vi "MethodSignatureDialogvi.vi"() -> (2 "Cancelled":bool)   [LabVIEW 2014, in "ClassWriterNative.lvclass"]
uses:
  <resource>/Framework/Providers/Open_GDS/ClassProviders/Provider_LvNativeClass/ClassWriterNative_class/ClassWriterNative.lvclass
  <resource>/Framework/Providers/Open_GDS/SubVIs/GOOP_HelpButton.ctl
panel:
  in  "_HelpCreateSignature":T1
  in  "_UpdateSignature":bool caption="Update this signature"
  in  "_InsertTag":bool caption="Insert tag"
  out "_TagPreview":string caption="Tag preview"
  in  "_SelectTagToAdd":T2(ring) caption="Select a tag to a cursor"
  in  "_SignatureName":string caption="Signature name"
  in  "_ModifySignature":bool caption="Modify signature"
  in  "_RemoveSignature":bool caption="Remove signature"
  in  "_Cancel":bool caption="Cancel"
  in  "_Done":bool caption="Done"
  in  "_AddSignature":bool caption="Add this signature"
  in  "_Signatures":i32[](listbox) caption="Signatures"
  in  "_SignatureText":string caption="Signature text"
  out "error out":errorcluster
  in  "error in":errorcluster
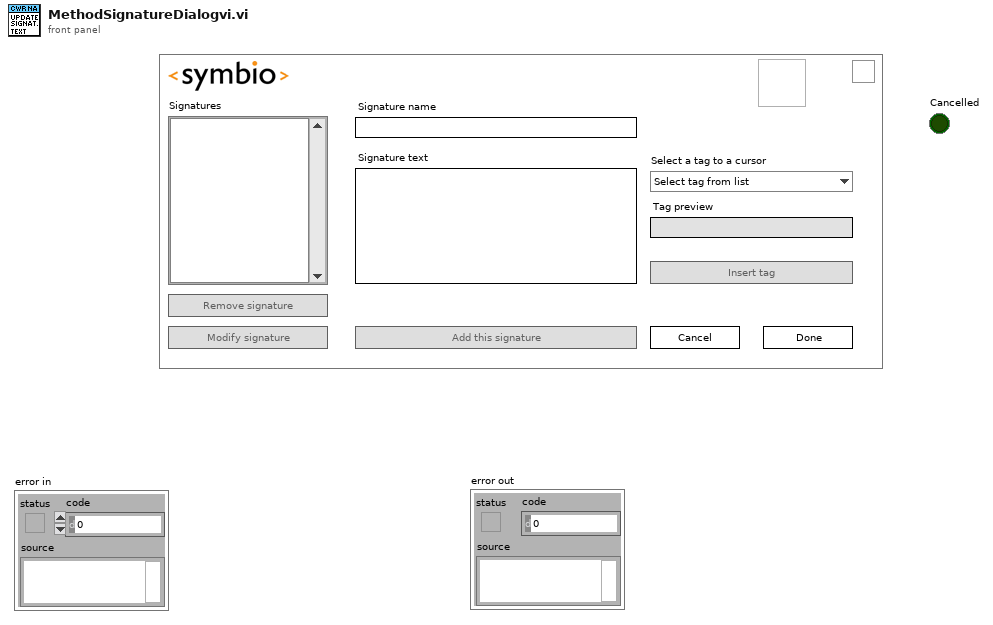
[diagram p1: front panel]
types:
  T1 = typedef "GOOP_HelpButton.ctl" = bool
  T2 = enum16{"Select tag from list", "<Date>", "<DateTime>", "<User>", "<LvVersion>"}
  T3 = cluster{"Cancelled":bool, "SignatureName":string[], "SignatureText":string[], "Current":i32}
  T4 = cluster{"SignatureName":string[], "SignatureText":string[], "Current":i32}
  T5 = cluster{"SignatureName":string[], "SignatureText":string[], i32}
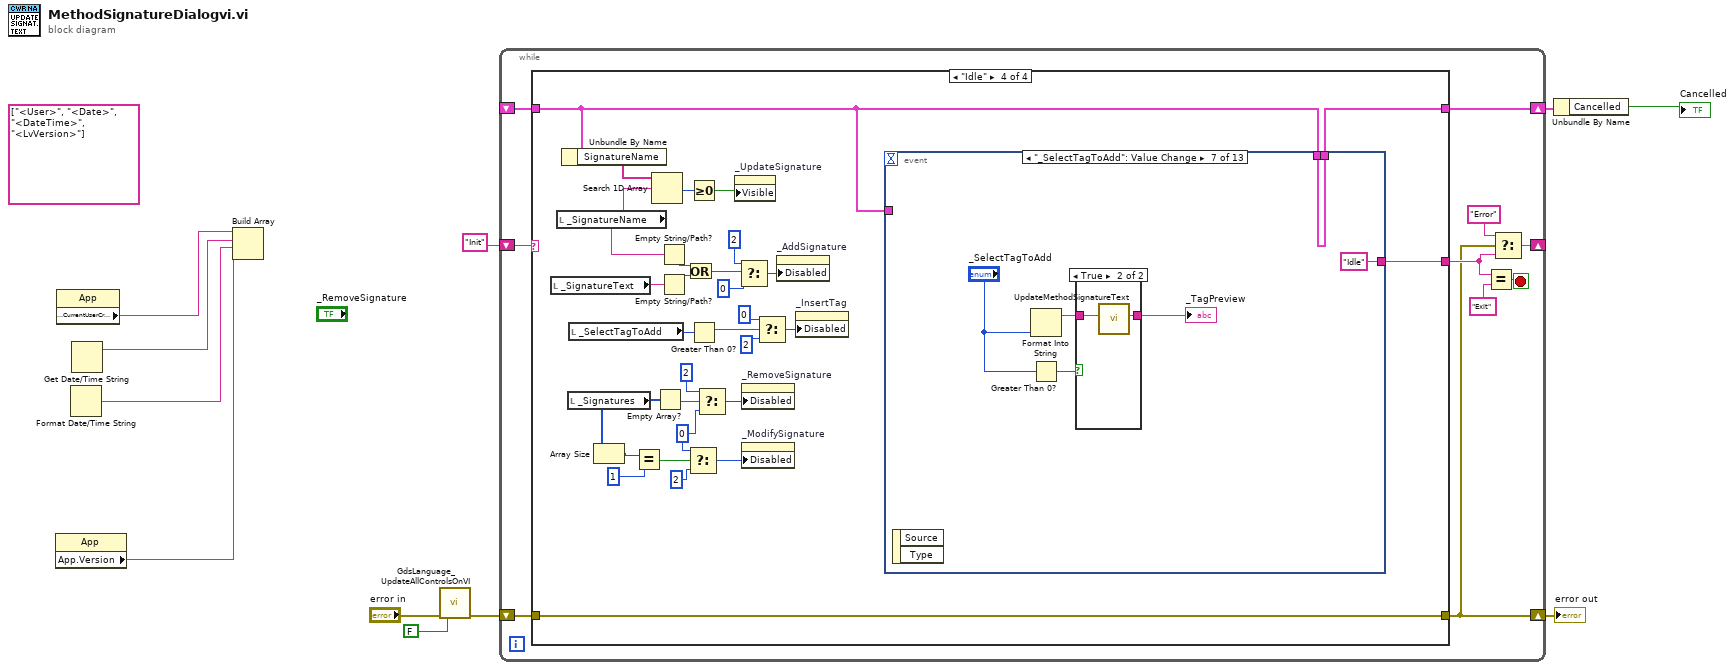
[diagram p0: block diagram]
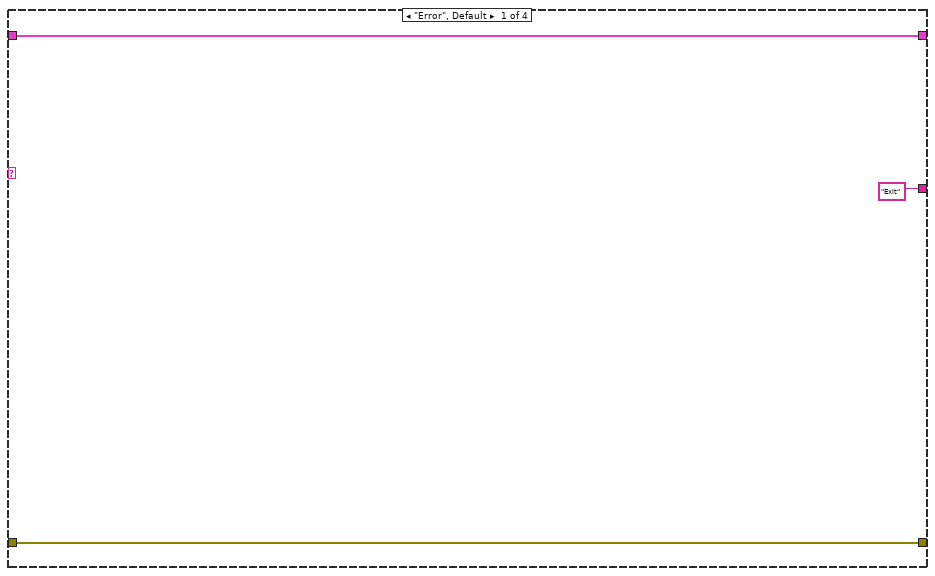
[diagram p2: hidden frame]
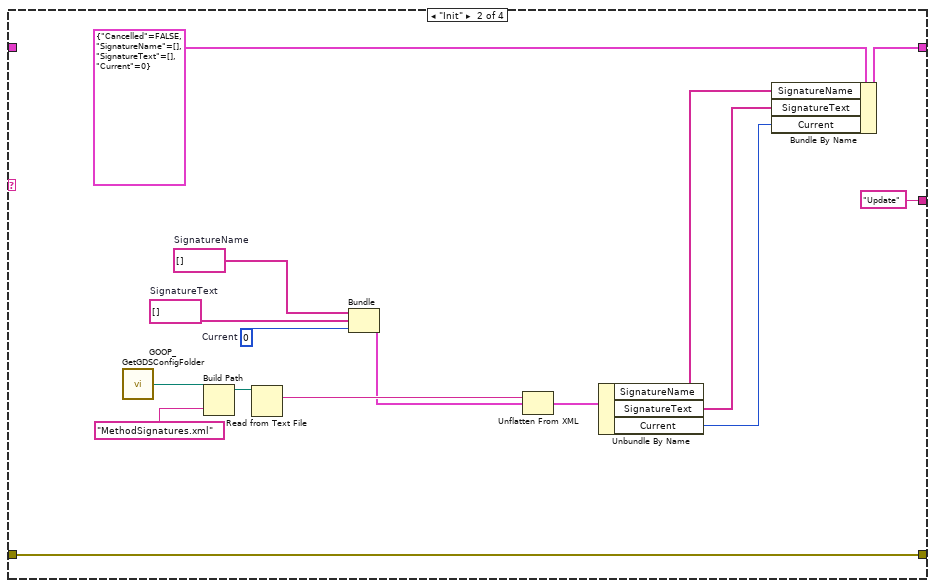
[diagram p3: hidden frame]
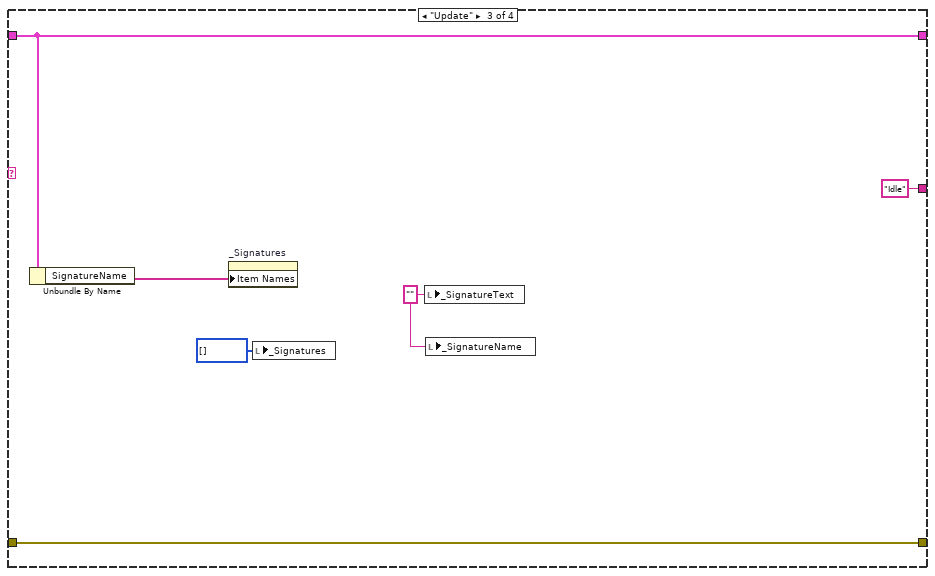
[diagram p4: hidden frame]
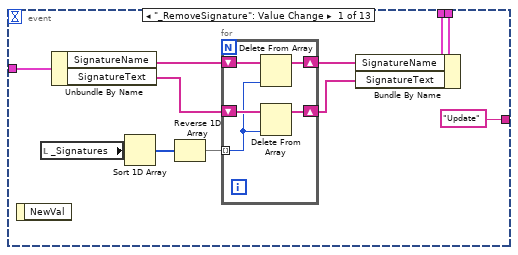
[diagram p5: hidden frame]
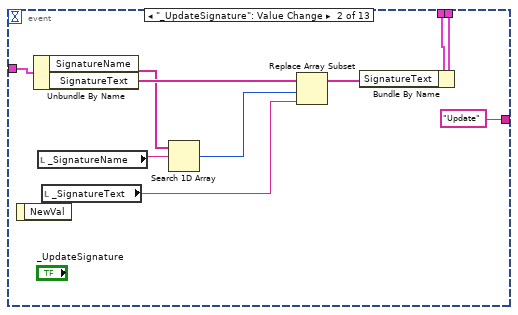
[diagram p6: hidden frame]
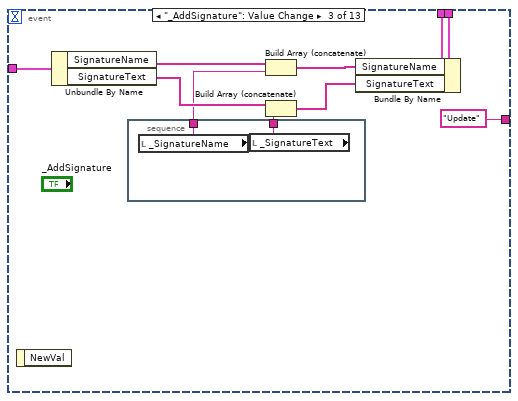
[diagram p7: hidden frame]
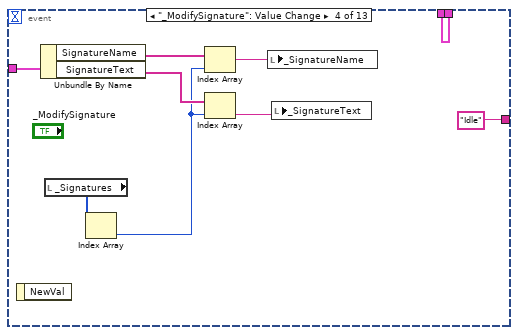
[diagram p8: hidden frame]
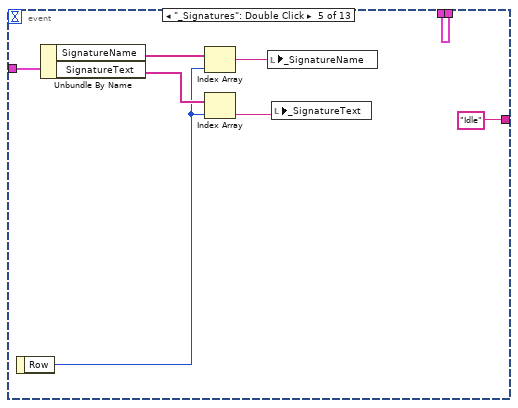
[diagram p9: hidden frame]
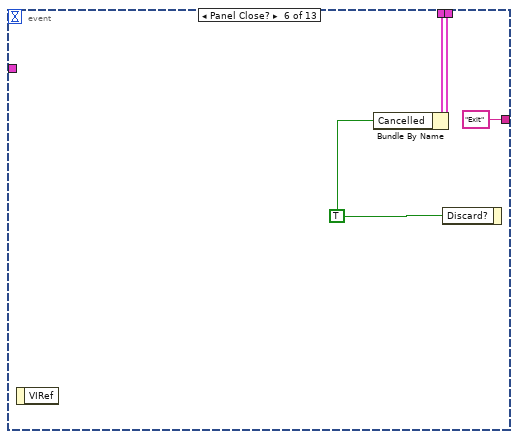
[diagram p10: hidden frame]
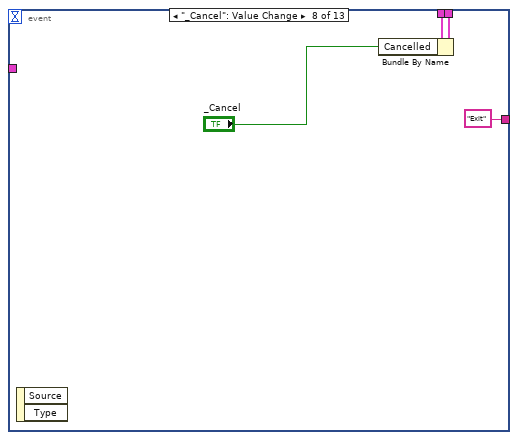
[diagram p12: hidden frame]
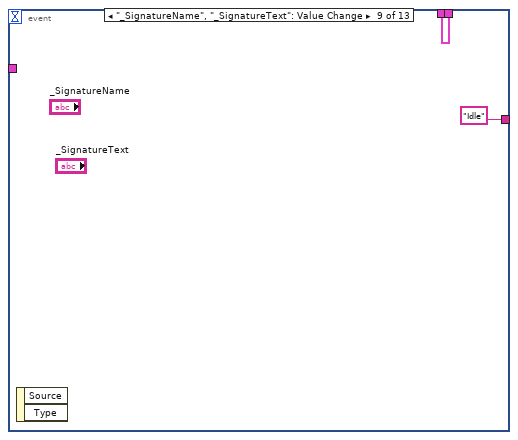
[diagram p13: hidden frame]
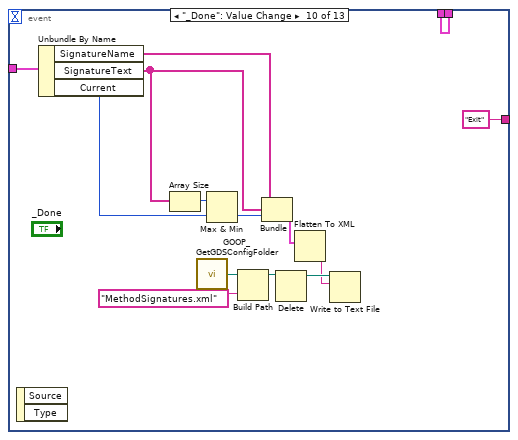
[diagram p14: hidden frame]
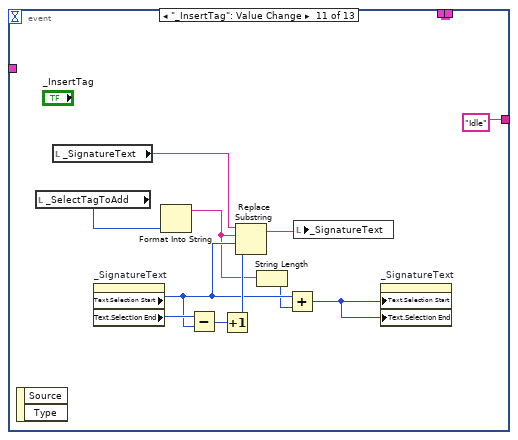
[diagram p15: hidden frame]
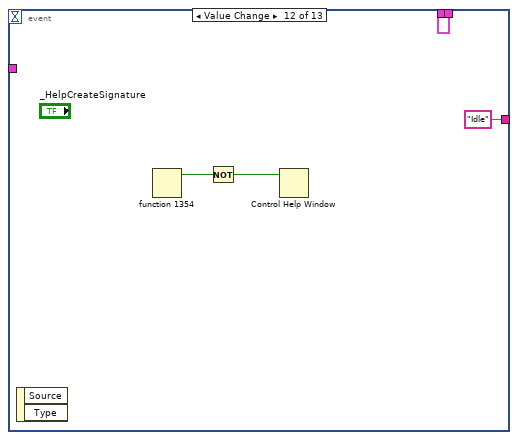
[diagram p16: hidden frame]
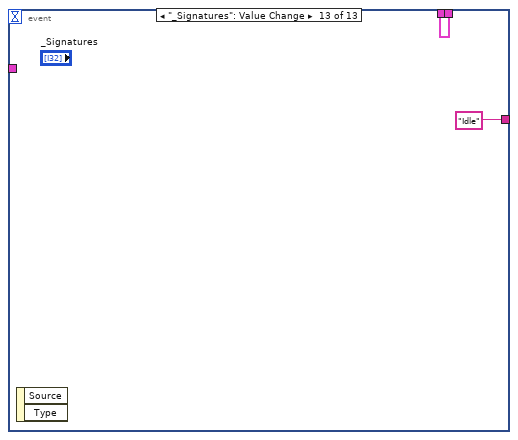
[diagram p17: hidden frame]
diagram:
  (unwired) string[] ["<User>", "<Date>", "<DateTime>", "<LvVersion>"]
  n1 = property class="App"() -> ("App.Version"=w8:string)  [unwired: 2 in, 2 out]
  n2 = property class="App"() -> ("App.CurrentUserCredential"=w11:string)  [unwired: 2 in, 2 out]
  n3 = Format Date/Time String() -> (date/time string=w9:string)  [unwired: 3 in]
  n4 = Get Date/Time String() -> (date string=w10:string)  [unwired: 3 in, 1 out]
  n5 = Build Array(w11, w10, w9, w8) -> ()  [unwired: 1 out]
  n6 = call <resource>:"GdsLanguage_UpdateAllControlsOnVI.vi"("error in (no error)"="error in", "CreateLanguageFile(Use this to create a languageFile)"=FALSE) -> ("error out"=w2:errorcluster)  [unwired: 16 in, 1 out]
  n7 = while {
    shift-right: [w14] -> w4
    shift-left: w2 -> [w21]
    shift-right: [w19] -> _
    shift-left: "Init" -> [w20]
    shift-right: [w13] -> w6
    shift-left: _ -> [w12]
    stop <- w18 stop-if-true
    n8 = case shown="\"Idle\"" w20 {
      tunnel: w21 -> [w24 w39 w44 w74]
      tunnel: [w24 w39 w44 w74] -> w14
      tunnel: ["Exit" "Update" "Idle" w75] -> w15
      tunnel: [w22 w37 w45 w76] -> w13
      tunnel: w12 -> [w22 _ w45 w63]
      frame "Error", Default {
      }
      frame "Init" {
        w32 = string[] []  # SignatureText
        w33 = string[] []  # SignatureName
        w30 = 0  # Current
        n9 = call <resource>:"GOOP_GetGDSConfigFolder.vi"() -> ("GDSFolderPath"=w36:path)
        n10 = Build Path(base path=w36, name or relative path="MethodSignatures.xml") -> (appended path=w35:path)
        n11 = Read from Text File(file (use dialog)=w35) -> (text=w34:string)  [unwired: 3 in, 3 out]
        n12 = Bundle("SignatureName"=w33, "SignatureText"=w32, "Current"=w30) -> (w31:T4)  [unwired: 1 in]
        n13 = Unflatten From XML(xml string=w34, type=w31) -> (value=w29:T4)  [unwired: 1 in, 1 out]
        n14 = Unbundle By Name(w29) -> ("SignatureName"=w28:string[], "SignatureText"=w27:string[], "Current"=w26:i32)
        n15 = Bundle By Name(cluster=T3 {"Cancelled"=FALSE, "SignatureName"=[], "SignatureText"=[], "Current"=0}, "SignatureName"=w28, "SignatureText"=w27, "Current"=w26) -> (w37:T3)
      }
      frame "Update" {
        w41 = "" ("_SignatureText")
        n16 = Unbundle By Name(w45) -> ("SignatureName"=w43:string[])
        n17 = property on="_Signatures" class="LstBox (strict)"("Item Names"=w43) -> ()  [unwired: 2 in, 2 out]
        n18 = local write "_Signatures"(i32[] [] ("_Signatures")) -> ()
        n19 = local write "_SignatureText"(w41) -> ()
        n20 = local write "_SignatureName"(w41) -> ()
      }
      frame "Idle" {
        w66 = u8 0 ("f")
        n21 = local read "_SignatureText"() -> (w58:string)
        n22 = local read "_SignatureName"() -> (w59:string)
        n23 = Unbundle By Name(w63) -> ("SignatureName"=w62:string[])
        n24 = local read "_Signatures"() -> (w70:i32[])
        n25 = local read "_SelectTagToAdd"() -> (w51:T2)
        n26 = Array Size(array=w70) -> (size(s)=w69:i32)
        n27 = Equal?(x=w69, y=1) -> (x = y?=w65:bool)
        n28 = Search 1D Array(1D array=w62, element=w59) -> (index of element=w61:i32)  [unwired: 1 in]
        n29 = Empty Array?(array=w70) -> (empty?=w73:bool)
        n30 = Empty String/Path?(string/path=w59) -> (empty?=w57:bool)
        n31 = Empty String/Path?(string/path=w58) -> (empty?=w56:bool)
        n32 = Or(x=w57, y=w56) -> (x .or. y?=w53:bool)
        n33 = Select(t=w66, s=w65, f=u8 2) -> (s? t:f=w64:u8)
        n34 = Greater Or Equal To 0?(x=w61) -> (x >= 0?=w60:bool)
        n35 = Greater Than 0?(x=w51) -> (x > 0?=w49:bool)
        n36 = Select(t=u8 2 ("Disabled"), s=w73, f=w66) -> (s? t:f=w72:u8)
        n37 = property on="_UpdateSignature" class="Bool"("Visible"=w60) -> ()  [unwired: 2 in, 2 out]
        n38 = Select(t=u8 2 ("Disabled"), s=w53, f=u8 0) -> (s? t:f=w52:u8)
        n39 = property on="_RemoveSignature" class="Bool"("Disabled"=w72) -> ()  [unwired: 2 in, 2 out]
        n40 = property on="_ModifySignature" class="Bool"("Disabled"=w64) -> ()  [unwired: 2 in, 2 out]
        n41 = Select(t=u8 0 ("f"), s=w49, f=u8 2) -> (s? t:f=w47:u8)
        n42 = property on="_AddSignature" class="Bool"("Disabled"=w52) -> ()  [unwired: 2 in, 2 out]
        n43 = property on="_InsertTag" class="Bool"("Disabled"=w47) -> ()  [unwired: 2 in, 2 out]
        n44 = event shown="[6] \"_SelectTagToAdd\": Value Change" {
          selector: _ -> [_ _ _ _ _ _ _ _ _ _ _ _ _]
          dyn-events: _ -> [_ _ _ _ _ _ _ _ _ _ _ _ _]
          timeout: _ -> [_ _ _ _ _ _ _ _ _ _ _ _ _]
          tunnel: w63 -> [w86 w101 w111 w115 w125 w134 w139 w147 w149 w163 w175 w177 w181]
          tunnel: [w85 w100 w110 w115 w125 w133 w139 w146 w149 w163 w175 w177 w181] -> w76
          tunnel: ["Update" "Update" "Update" "Idle" "Idle" "Exit" "Idle" "Exit" "Idle" "Exit" "Idle" "Idle" "Idle"] -> w75
          tunnel: w63 -> [w84 w99 w109 w122 w131 _ _ _ _ w162 _ _ _]
          event "_RemoveSignature": Value Change {
            n45 = event-data() -> ()  [unwired: 1 in, 1 out]
            n46 = local read "_Signatures"() -> (w79:i32[])
            n47 = Unbundle By Name(w84) -> ("SignatureName"=w83:string[], "SignatureText"=w81:string[])
            n48 = Sort 1D Array(array=w79) -> (sorted array=w78:i32[])
            n49 = Reverse 1D Array(array=w78) -> (reversed array=w77:i32[])
            n50 = for {
              tunnel: w77 -> [w88] mode=indexing
              shift-right: [w89] -> w80
              shift-left: w81 -> [w90]
              shift-right: [w91] -> w82
              shift-left: w83 -> [w92]
              n51 = Delete From Array(array=w92, index=w88) -> (array with subset deleted=w91:string[])  [unwired: 1 in, 1 out]
              n52 = Delete From Array(array=w90, index=w88) -> (array with subset deleted=w89:string[])  [unwired: 1 in, 1 out]
            }
            n53 = Bundle By Name(cluster=w86, "SignatureName"=w82, "SignatureText"=w80) -> (w85:T3)
          }
          event "_UpdateSignature": Value Change {
            n54 = event-data() -> ()  [unwired: 1 in, 1 out]
            n55 = Unbundle By Name(w99) -> ("SignatureName"=w96:string[], "SignatureText"=w98:string[])
            n56 = local read "_SignatureName"() -> (w95:string)
            n57 = local read "_SignatureText"() -> (w93:string)
            n58 = Search 1D Array(1D array=w96, element=w95) -> (index of element=w94:i32)  [unwired: 1 in]
            n59 = Replace Array Subset(array=w98, new element=w93, index=w94) -> (w97:string[])
            n60 = Bundle By Name(cluster=w101, "SignatureText"=w97) -> (w100:T3)
          }
          event "_AddSignature": Value Change {
            n61 = event-data() -> ()  [unwired: 1 in, 1 out]
            n62 = Unbundle By Name(w109) -> ("SignatureName"=w108:string[], "SignatureText"=w106:string[])
            n63 = stacked-sequence {
              tunnel: [w114] -> w104
              tunnel: [w113] -> w103
              frame #0 {
                n64 = local read "_SignatureName"() -> (w114:string)
                n65 = local read "_SignatureText"() -> (w113:string)
              }
            }
            n66 = Build Array (concatenate)(w108, w104) -> (w107:string[])
            n67 = Build Array (concatenate)(w106, w103) -> (w105:string[])
            n68 = Bundle By Name(cluster=w111, "SignatureName"=w107, "SignatureText"=w105) -> (w110:T3)
          }
          event "_ModifySignature": Value Change {
            n69 = event-data() -> ()  [unwired: 1 in, 1 out]
            n70 = Unbundle By Name(w122) -> ("SignatureName"=w121:string[], "SignatureText"=w120:string[])
            n71 = local read "_Signatures"() -> (w123:i32[])
            n72 = Index Array(array=w123) -> (element=w119:i32)  [unwired: 1 in]
            n73 = Index Array(array=w121, index=w119) -> (element=w117:string)
            n74 = Index Array(array=w120, index=w119) -> (element=w118:string)
            n75 = local write "_SignatureName"(w117) -> ()
            n76 = local write "_SignatureText"(w118) -> ()
          }
          event "_Signatures": Double Click {
            n77 = event-data() -> ("Row"=w124:i32)  [unwired: 1 in]
            n78 = Unbundle By Name(w131) -> ("SignatureName"=w130:string[], "SignatureText"=w129:string[])
            n79 = Index Array(array=w130, index=w124) -> (element=w127:string)
            n80 = Index Array(array=w129, index=w124) -> (element=w128:string)
            n81 = local write "_SignatureName"(w127) -> ()
            n82 = local write "_SignatureText"(w128) -> ()
          }
          event Panel Close? {
            w132 = TRUE ("Discard?")
            n83 = event-data() -> ()  [unwired: 1 in, 1 out]
            n84 = Bundle By Name(cluster=w134, "Cancelled"=w132) -> (w133:T3)
            n85 = event-data("Discard?"=w132) -> ()  [unwired: 1 in, 1 out]
          }
          event "_SelectTagToAdd": Value Change {
            n86 = event-data() -> ()  [unwired: 1 in, 2 out]
            n87 = Format Into String("_SelectTagToAdd") -> (resulting string=w141:string)  [unwired: 3 in, 1 out]
            n88 = Greater Than 0?(x="_SelectTagToAdd") -> (x > 0?=w136:bool)
            n89 = case shown="True" w136 {
              tunnel: w141 -> [_ w143]
              tunnel: [_ w142] -> w140
              frame False {
              }
              frame True {
                n90 = call <resource>:"UpdateMethodSignatureText.vi"("TagCodedStringIn"=w143) -> ("StringOut"=w142:string)  [unwired: 10 in]
              }
            }
            "_TagPreview" <- w140
          }
          event "_Cancel": Value Change {
            n91 = event-data() -> ()  [unwired: 1 in, 2 out]
            n92 = Bundle By Name(cluster=w147, "Cancelled"="_Cancel") -> (w146:T3)
          }
          event "_SignatureName", "_SignatureText": Value Change {
            n93 = event-data() -> ()  [unwired: 1 in, 2 out]
          }
          event "_Done": Value Change {
            n94 = event-data() -> ()  [unwired: 1 in, 2 out]
            n95 = Unbundle By Name(w162) -> ("SignatureName"=w159:string[], "SignatureText"=w157:string[], "Current"=w156:i32)
            n96 = Array Size(array=w157) -> (size(s)=w158:i32)
            n97 = call <resource>:"GOOP_GetGDSConfigFolder.vi"() -> ("GDSFolderPath"=w160:path)
            n98 = Max & Min(x=w158, y=w156) -> (min(x,y)=w155:i32)  [unwired: 1 out]
            n99 = Build Path(base path=w160, name or relative path="MethodSignatures.xml") -> (appended path=w153:path)
            n100 = Bundle("SignatureName"=w159, "SignatureText"=w157, w155) -> (w154:T5)  [unwired: 1 in]
            n101 = Delete(path (use dialog)=w153) -> (deleted path=w152:path)  [unwired: 4 in, 2 out]
            n102 = Flatten To XML(anything=w154) -> (xml string=w151:string)
            n103 = Write to Text File(file (use dialog)=w152, text=w151) -> ()  [unwired: 2 in, 3 out]
          }
          event "_InsertTag": Value Change {
            n104 = event-data() -> ()  [unwired: 1 in, 2 out]
            n105 = local read "_SelectTagToAdd"() -> (w169:T2)
            n106 = local read "_SignatureText"() -> (w173:string)
            n107 = property on="_SignatureText" class="Str"() -> ("Text.Selection Start"=w167:u32, "Text.Selection End"=w172:u32)  [unwired: 2 in, 2 out]
            n108 = Format Into String(w169) -> (resulting string=w166:string)  [unwired: 3 in, 1 out]
            n109 = Subtract(x=w172, y=w167) -> (x-y=w171:u32)
            n110 = Increment(x=w171) -> (x+1=w170:u32)
            n111 = Replace Substring(2:w170, 3:w167, 4:w166, 5:w173) -> (1:w168:string)  [unwired: 1 out]
            n112 = String Length(string=w166) -> (length=w165:i32)
            n113 = Add(x=w167, y=w165) -> (x+y=w164:u32)
            n114 = local write "_SignatureText"(w168) -> ()
            n115 = property on="_SignatureText" class="Str"("Text.Selection Start"=w164, "Text.Selection End"=w164) -> ()  [unwired: 2 in, 2 out]
          }
          event Value Change {
            n116 = event-data() -> ()  [unwired: 1 in, 2 out]
            n117 = fn#1354() -> (1:w179:bool)  [unwired: 1 out]
            n118 = Not(x=w179) -> (.not. x?=w178:bool)
            n119 = Control Help Window(1:w178) -> ()  [unwired: 1 in]
          }
          event "_Signatures": Value Change {
            n120 = event-data() -> ()  [unwired: 1 in, 2 out]
          }
        }
      }
    }
    n121 = Equal?(x=w15, y="Exit") -> (x = y?=w18:bool)
    n122 = Select(t="Error", s=w14, f=w15) -> (s? t:f=w19:string)
  }
  "error out" <- w4
  n123 = Unbundle By Name(w6) -> ("Cancelled"=→"Cancelled":bool)
